vi "Complex FIR Filter (complex signal).vi"(2 "init/cont (init:F)":bool, 3 "FIR Coefficients":cdb[](array[numeric]), 5 "X":cdb[](array[numeric])) -> (0 "error":i32, 1 "Filtered X":cdb[](array[numeric]))   [LabVIEW 2017, in "NI_AALBase.lvlib"]
uses:
  <vilib>/Analysis/NI_AALBase.lvlib
  <resource>/lvanlys.dll
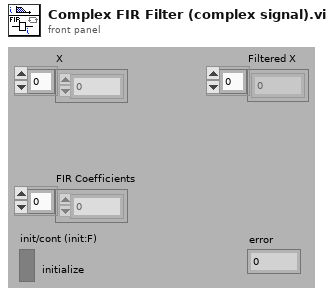
[diagram p1: front panel]
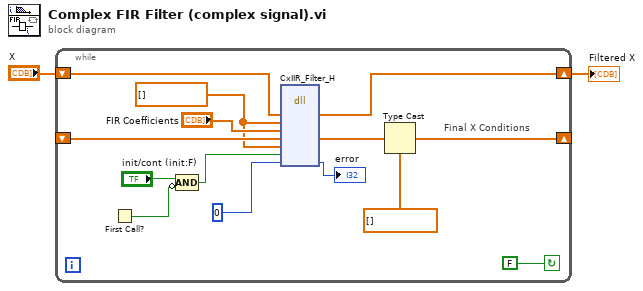
[diagram p0: block diagram]
diagram:
  n1 = while {
    shift-left: _ -> [w4]
    shift-right: [w16] -> _
    shift-right: [w7] -> w1
    shift-left: "X" -> [w8]
    stop <- FALSE continue-if-true
    w3 = cdb[] [] ("Reverse Coefficients")
    # "Final X Conditions"
    n2 = First Call?() -> (First Call?: T/F=w5:bool)
    n3 = Compound Arithmetic op=AND("init/cont (init:F)", invert w5) -> (w6:bool)
    n4 = dll-call lib="e:/builds/penguin/labview/branches/2017/dev/dist/resource/lvanlys.*" fn="CxIIR_Filter_H"("X"=w8, "Reverse Coefficients"=w3, "FIR Coefficients"="FIR Coefficients", "type for the shift register"=w4, "Reverse Coefficients"=w3, w6, "dsperr"=0) -> ("X"=w7:cdb[], "type for the shift register"=w11:cdb[], "dsperr"=→"error":i32)  [unwired: 8 in, 2 out]
    n5 = Type Cast(type=cdb[] [] ("type for the shift register"), x=w11) -> (*(type *) &x=w16:cdb[])
  }
  "Filtered X" <- w1
